vi "Voltage Min Read.vi"   [LabVIEW 2023, in "Cycler.lvclass"]
uses:
  Cycler.lvclass
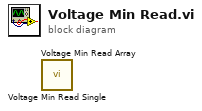
[diagram p0: block diagram]
diagram:
  n1 = call "Voltage Min Read Single.vi"() -> ()  [unwired: 8 in, 4 out]
  n2 = call "Voltage Min Read Array.vi"() -> ()  [unwired: 8 in, 4 out]
